vi "GUI_Final_PID.vi"() -> ()   [LabVIEW 2013]
uses:
  <vilib>/Instr/_visa.llb/VISA Configure Serial Port (Instr).vi
panel:
  in  "Send to encoder":bool
  out "Angle":u8[](array[numeric])
  out "Left":bool
  out "Right":bool
  out "read buffer":string
  in  "Stop":bool
  in  "Angle":string
  out "Error":errorcluster
  out "Arduino Data":string
  in  "Mode":bool
  in  "Baud Rate 2":u32=9600
  in  "Port 2":refnum<visa-resource-name>
  in  "Baud Rate":u32=9600
  in  "Port":refnum<visa-resource-name>
  out "Response 2":string
  in  "Command":string
  out "error out":errorcluster
  out "Numeric 12":i32
  in  "angle":i32
  in  "OK":bool
  in  "Commands":string(combo)
  out "error out 2":errorcluster
  in  "MODE":bool
  # "Arduino Interface"
  # "Encoder Interface"
  # "Text Mode"
  # "Button Mode"
  # "Select : ON : Text Mode , \n              OFF : ButtonMode"
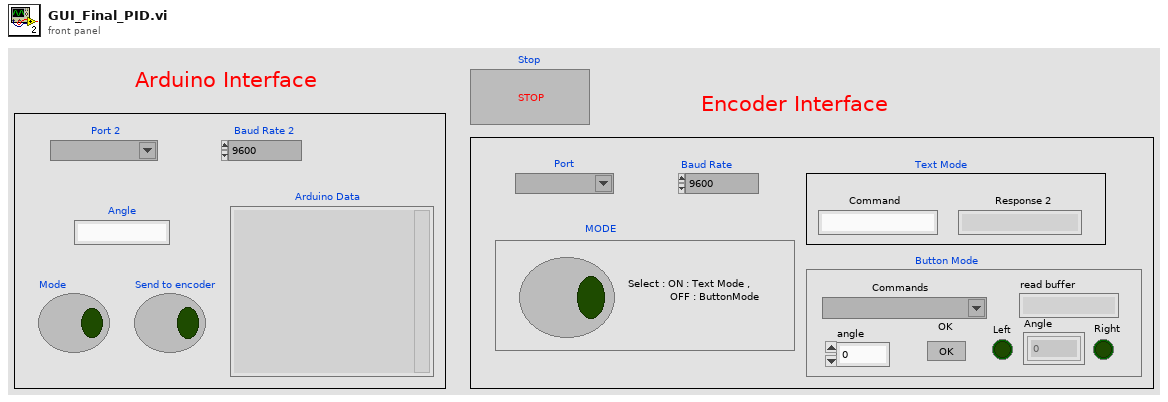
[diagram p1: front panel]
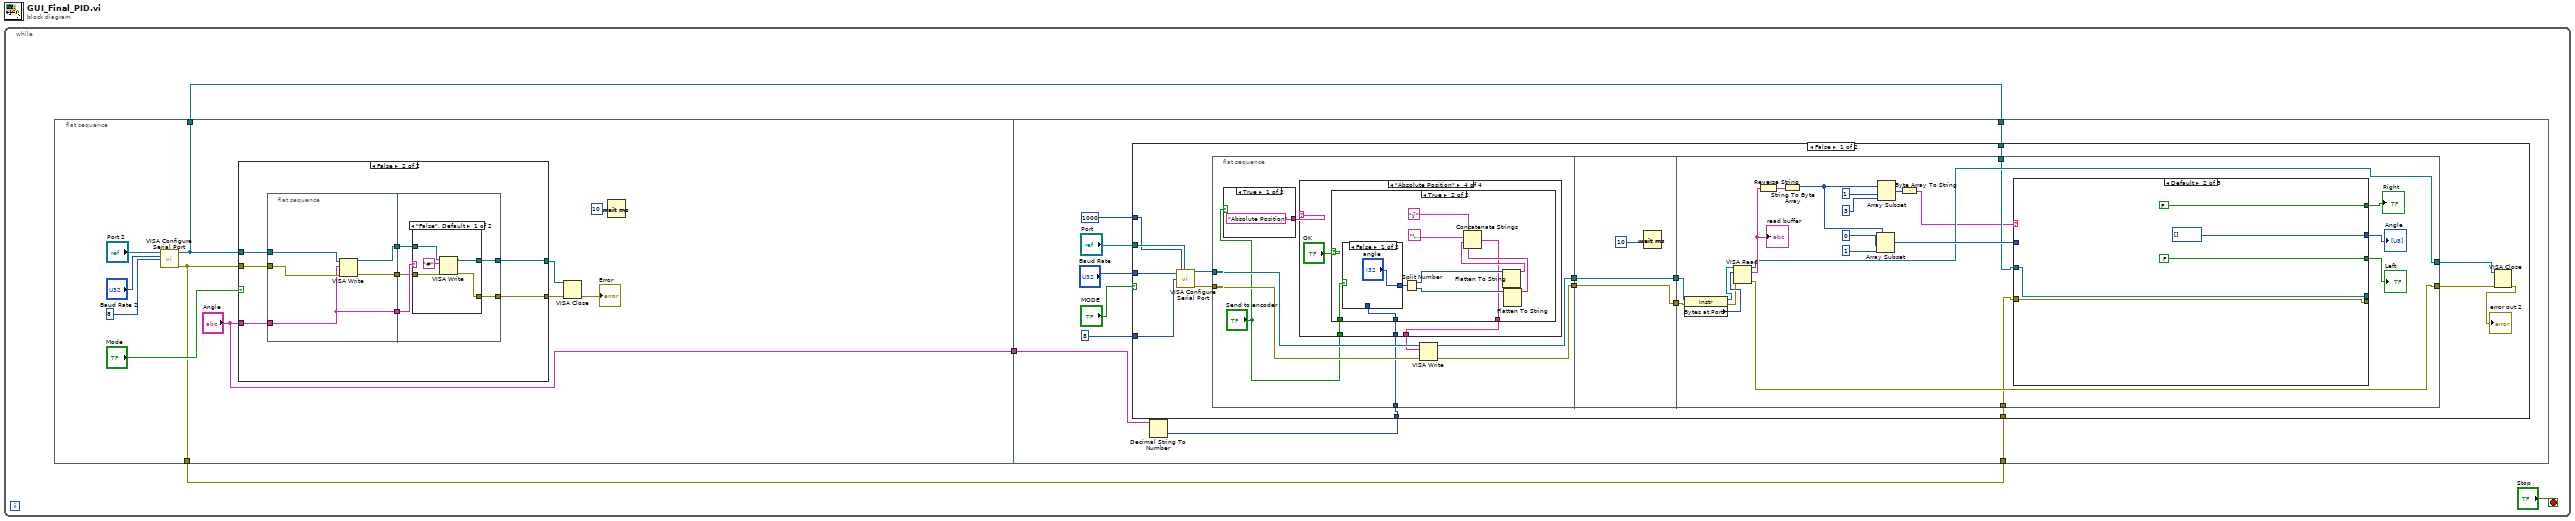
[diagram p0: block diagram]
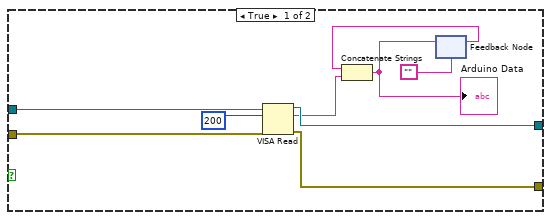
[diagram p2: hidden frame]
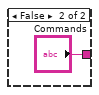
[diagram p4: hidden frame]
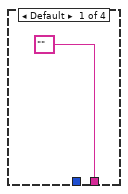
[diagram p5: hidden frame]
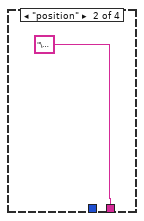
[diagram p6: hidden frame]
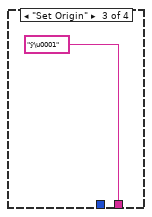
[diagram p7: hidden frame]
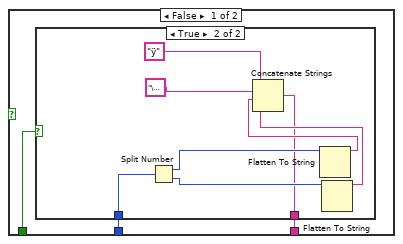
[diagram p8: hidden frame]
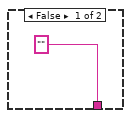
[diagram p9: hidden frame]
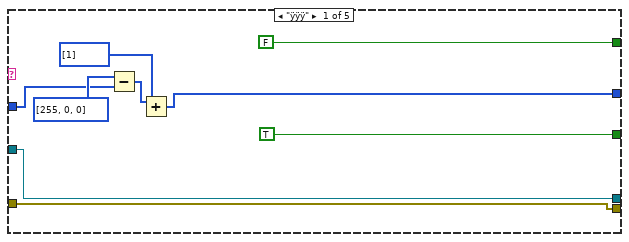
[diagram p11: hidden frame]
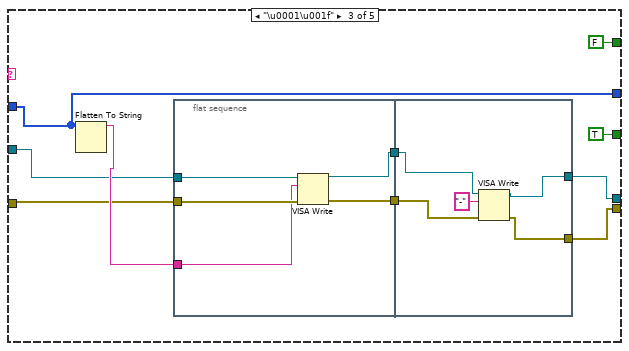
[diagram p12: hidden frame]
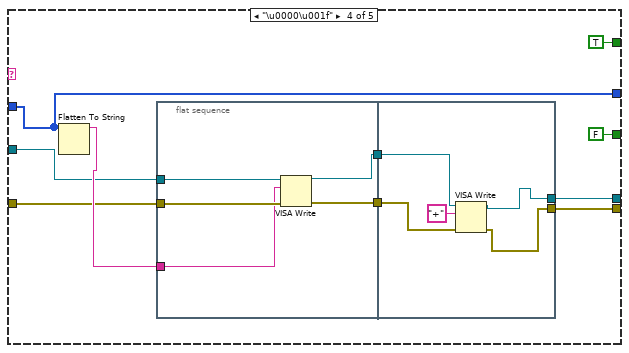
[diagram p13: hidden frame]
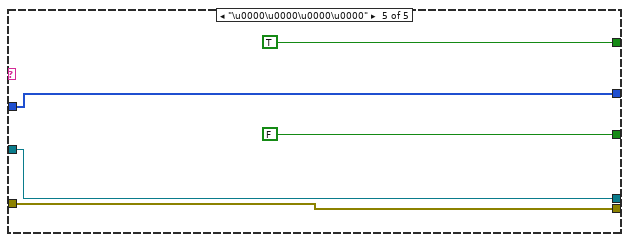
[diagram p14: hidden frame]
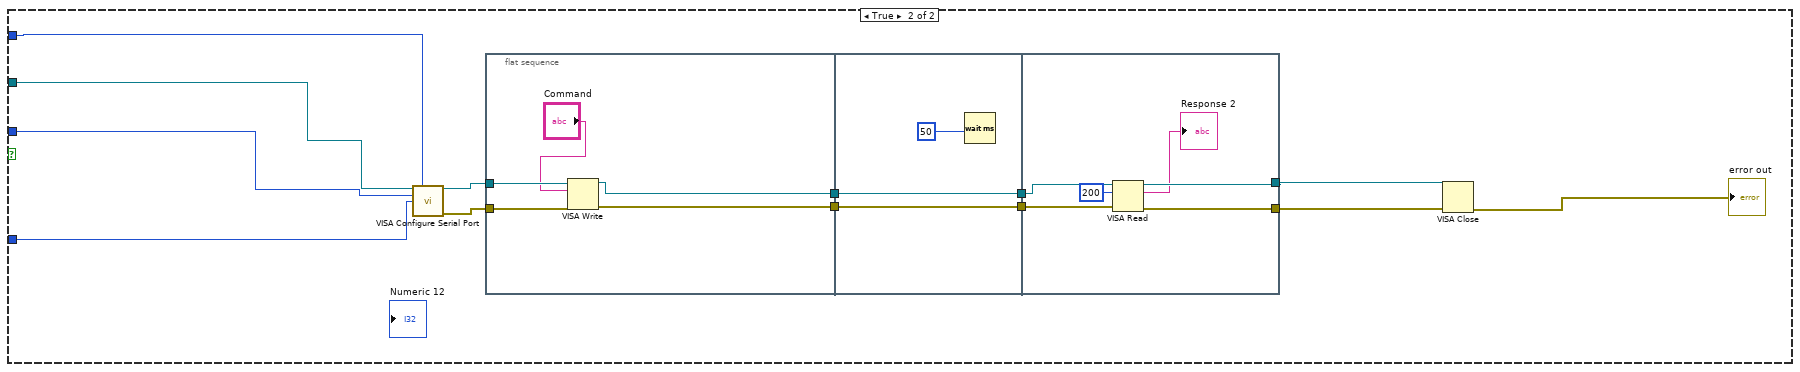
[diagram p15: hidden frame]
diagram:
  n1 = while {
    stop <- "Stop" stop-if-true
    n2 = flat-sequence {
      tunnel: ["Angle"] -> w4
      tunnel: [w6] -> w2
      tunnel: [w5] -> w1
      tunnel: w4 -> [w54]
      tunnel: w2 -> [w51]
      tunnel: w1 -> [w50]
      frame #0 {
        n3 = call-poly "VISA Configure Serial Port"("VISA resource name"="Port 2", "baud rate (9600)"="Baud Rate 2", "data bits (8)"=u16 8) -> ("VISA resource name out"=w6:refnum<visa-resource-name>, "error out"=w5:errorcluster)  [unwired: 11 in]
        n4 = case shown="False" "Mode" {
          tunnel: w6 -> [w22 w32]
          tunnel: [w23 w26] -> w14
          tunnel: [w24 w27] -> w15
          tunnel: w5 -> [w21 w31]
          tunnel: "Angle" -> [_ w25]
          frame True {
            n5 = VISA Read(VISA resource name=w22, byte count=u32 200, error in (no error)=w21) -> (VISA resource name out=w24:refnum<visa-resource-name>, read buffer=w19:string, error out=w23:errorcluster)  [unwired: 1 out]
            n6 = feedback #1("") -> (w18:string)
            n7 = Concatenate Strings(w18, w19) -> (w17:string)
            "Arduino Data" <- w17
            n8 = feedback-in #1(w17) -> ()
          }
          frame False {
            n9 = flat-sequence {
              tunnel: w32 -> [w37]
              tunnel: w31 -> [w36]
              tunnel: [w33] -> w30
              tunnel: [w35] -> w29
              tunnel: [w34] -> w28
              tunnel: w25 -> [w33]
              tunnel: w30 -> [w42]
              tunnel: w29 -> [w41]
              tunnel: w28 -> [w40]
              tunnel: [w39] -> w27
              tunnel: [w38] -> w26
              frame #0 {
                n10 = VISA Write(VISA resource name=w37, write buffer=w33, error in (no error)=w36) -> (VISA resource name out=w35:refnum<visa-resource-name>, error out=w34:errorcluster)  [unwired: 1 out]
              }
              frame #1 {
                n11 = case shown="\"False\", Default" w42 {
                  tunnel: w41 -> [w46 w49]
                  tunnel: w40 -> [w45 w48]
                  tunnel: [w44 w49] -> w39
                  tunnel: [w43 w48] -> w38
                  frame "False", Default {
                    n12 = VISA Write(VISA resource name=w46, write buffer="#", error in (no error)=w45) -> (VISA resource name out=w44:refnum<visa-resource-name>, error out=w43:errorcluster)  [unwired: 1 out]
                  }
                  frame "" {
                  }
                }
              }
            }
          }
        }
        n13 = VISA Close(VISA resource name=w15, error in (no error)=w14) -> (error out=→"Error":errorcluster)
        n14 = Wait (ms)(milliseconds to wait=u32 10) -> ()  [unwired: 1 out]
      }
      frame #1 {
        n15 = Decimal String To Number(string=w54) -> (number=w52:i32)  [unwired: 2 in, 1 out]
        n16 = case shown="False" "MODE" {
          tunnel: u32 1000 ("timeout (10sec)") -> [w63 w203]
          tunnel: "Port" -> [w68 w202]
          tunnel: "Baud Rate" -> [w67 w201]
          tunnel: u16 8 ("data bits (8)") -> [w65 w200]
          tunnel: w52 -> [w64 _]
          tunnel: w51 -> [w60 _]
          tunnel: w50 -> [w59 _]
          frame False {
            n17 = call-poly "VISA Configure Serial Port"("VISA resource name"=w68, "timeout (10sec)"=w63, "baud rate (9600)"=w67, "data bits (8)"=w65) -> ("VISA resource name out"=w72:refnum<visa-resource-name>, "error out"=w71:errorcluster)  [unwired: 10 in]
            n18 = flat-sequence {
              tunnel: [w81] -> w74
              tunnel: w72 -> [w80]
              tunnel: w71 -> [w79]
              tunnel: [w82] -> w70
              tunnel: w64 -> [w76]
              tunnel: [w117] -> w73
              tunnel: w74 -> [w116]
              tunnel: w70 -> [w117]
              tunnel: [w116] -> w69
              tunnel: w73 -> [w133]
              tunnel: w69 -> [w139]
              tunnel: [w123] -> w62
              tunnel: [w122] -> w61
              tunnel: w60 -> [w121]
              tunnel: w59 -> [w120]
              frame #0 {
                n19 = case shown="True" "Send to encoder" {
                  tunnel: ["Absolute Position" ("Commands") "Commands"] -> w78
                  frame True {
                  }
                  frame False {
                  }
                }
                n20 = case shown="\"Absolute Position\"" w78 {
                  tunnel: ["" "\u001f" "ÿ\u0001" w89] -> w77
                  tunnel: w76 -> [_ _ _ w90]
                  tunnel: "Send to encoder" -> [_ _ _ w88]
                  frame Default {
                  }
                  frame "position" {
                  }
                  frame "Set Origin" {
                  }
                  frame "Absolute Position" {
                    n21 = case shown="True" "OK" {
                      tunnel: w90 -> [w94 w105]
                      tunnel: [w93 w106] -> w89
                      tunnel: w88 -> [w92 w104]
                      frame False {
                        n22 = case shown="True" w92 {
                          tunnel: w94 -> [_ w97]
                          tunnel: ["" w96] -> w93
                          frame False {
                          }
                          frame True {
                            n23 = Split Number(x=w97) -> (hi(x)=w99:u16, lo(x)=w98:u16)
                            n24 = Flatten To String(anything=w99) -> (data string=w101:string)  [unwired: 3 in, 2 out]
                            n25 = Flatten To String(anything=w98) -> (data string=w100:string)  [unwired: 3 in, 2 out]
                            n26 = Concatenate Strings("ÿ" ("string"), "\u0002" ("string"), w101, w100) -> (w96:string)
                          }
                        }
                      }
                      frame True {
                        n27 = case shown="False" w104 {
                          tunnel: w105 -> [_ w115]
                          tunnel: ["angle" w115] -> w107
                          frame False {
                          }
                          frame True {
                          }
                        }
                        n28 = Split Number(x=w107) -> (hi(x)=w109:u16, lo(x)=w108:u16)
                        n29 = Flatten To String(anything=w109) -> (data string=w111:string)  [unwired: 3 in, 2 out]
                        n30 = Flatten To String(anything=w108) -> (data string=w110:string)  [unwired: 3 in, 2 out]
                        n31 = Concatenate Strings("ÿ" ("string"), "\u0002" ("string"), w111, w110) -> (w106:string)
                      }
                    }
                  }
                }
                n32 = VISA Write(VISA resource name=w80, write buffer=w77, error in (no error)=w79) -> (VISA resource name out=w82:refnum<visa-resource-name>, error out=w81:errorcluster)  [unwired: 1 out]
              }
              frame #1 {
                n33 = Wait (ms)(milliseconds to wait=u32 10) -> ()  [unwired: 1 out]
              }
              frame #2 {
                n34 = property class="Instr"(reference=w133, error in=w139) -> (reference out=w132:refnum<visa-resource-name>, error out=w138:errorcluster, "Bytes at Port"=w140:u32)
                n35 = VISA Read(VISA resource name=w132, byte count=w140, error in (no error)=w138) -> (VISA resource name out=w123:refnum<visa-resource-name>, read buffer=w135:string, error out=w122:errorcluster)  [unwired: 1 out]
                "read buffer" <- w135
                n36 = Reverse String(1:w135) -> (0:w131:string)
                n37 = String To Byte Array(string=w131) -> (unsigned byte array=w137:u8[])
                n38 = Array Subset(array=w137, index=0, length=1) -> (w124:u8[])
                n39 = Array Subset(array=w137, index=1, length=3) -> (w134:u8[])
                n40 = Byte Array To String(unsigned byte array=w134) -> (string=w119:string)
                n41 = case shown="Default" w119 {
                  tunnel: [w146 u8[] [] w155 w175 w195] -> w126
                  tunnel: [TRUE ("Boolean") FALSE ("Boolean") TRUE ("Boolean") FALSE ("Boolean") FALSE ("Boolean")] -> w125
                  tunnel: [FALSE ("Boolean") FALSE ("Boolean") FALSE ("Boolean") TRUE ("Boolean") TRUE ("Boolean")] -> w127
                  tunnel: w120 -> [w143 w151 w158 w179 w197]
                  tunnel: [w142 w150 w157 w178 w196] -> _
                  tunnel: [w143 w151 w156 w177 w197] -> _
                  tunnel: w121 -> [w142 w150 w159 w176 w196]
                  tunnel: w124 -> [w141 _ w155 w175 w195]
                  frame "ÿÿÿ" {
                    n42 = Subtract(x=u8[] [255, 0, 0] ("y"), y=w141) -> (x-y=w149:u8[])
                    n43 = Add(x=w149, y=u8[] [1]) -> (x+y=w146:u8[])
                  }
                  frame Default {
                  }
                  frame "\u0001\u001f" {
                    n44 = Flatten To String(anything=w155) -> (data string=w160:string)  [unwired: 3 in, 2 out]
                    n45 = flat-sequence {
                      tunnel: [w169] -> w162
                      tunnel: [w168] -> w161
                      tunnel: w159 -> [w167]
                      tunnel: w158 -> [w166]
                      tunnel: w160 -> [w165]
                      tunnel: w162 -> [w173]
                      tunnel: w161 -> [w172]
                      tunnel: [w171] -> w157
                      tunnel: [w170] -> w156
                      frame #0 {
                        n46 = VISA Write(VISA resource name=w167, write buffer=w165, error in (no error)=w166) -> (VISA resource name out=w169:refnum<visa-resource-name>, error out=w168:errorcluster)  [unwired: 1 out]
                      }
                      frame #1 {
                        n47 = VISA Write(VISA resource name=w173, write buffer="-", error in (no error)=w172) -> (VISA resource name out=w171:refnum<visa-resource-name>, error out=w170:errorcluster)  [unwired: 1 out]
                      }
                    }
                  }
                  frame "\u0000\u001f" {
                    n48 = Flatten To String(anything=w175) -> (data string=w180:string)  [unwired: 3 in, 2 out]
                    n49 = flat-sequence {
                      tunnel: [w189] -> w182
                      tunnel: [w188] -> w181
                      tunnel: w176 -> [w187]
                      tunnel: w179 -> [w186]
                      tunnel: w180 -> [w185]
                      tunnel: w182 -> [w192]
                      tunnel: w181 -> [w193]
                      tunnel: [w191] -> w178
                      tunnel: [w190] -> w177
                      frame #0 {
                        n50 = VISA Write(VISA resource name=w187, write buffer=w185, error in (no error)=w186) -> (VISA resource name out=w189:refnum<visa-resource-name>, error out=w188:errorcluster)  [unwired: 1 out]
                      }
                      frame #1 {
                        n51 = VISA Write(VISA resource name=w192, write buffer="+", error in (no error)=w193) -> (VISA resource name out=w191:refnum<visa-resource-name>, error out=w190:errorcluster)  [unwired: 1 out]
                      }
                    }
                  }
                  frame "\u0000\u0000\u0000\u0000" {
                  }
                }
                "Left" <- w125
                "Right" <- w127
                "Angle" <- w126
              }
            }
            n52 = VISA Close(VISA resource name=w62, error in (no error)=w61) -> (error out=→"error out 2":errorcluster)
          }
          frame True {
            n53 = call-poly "VISA Configure Serial Port"("VISA resource name"=w202, "timeout (10sec)"=w203, "baud rate (9600)"=w201, "data bits (8)"=w200) -> ("VISA resource name out"=w208:refnum<visa-resource-name>, "error out"=w207:errorcluster)  [unwired: 10 in]
            n54 = flat-sequence {
              tunnel: w208 -> [w215]
              tunnel: w207 -> [w217]
              tunnel: [w214] -> w212
              tunnel: [w216] -> w211
              tunnel: [w219] -> w210
              tunnel: w212 -> [w219]
              tunnel: [w218] -> w209
              tunnel: w211 -> [w218]
              tunnel: w210 -> [w226]
              tunnel: w209 -> [w225]
              tunnel: [w224] -> w205
              tunnel: [w223] -> w206
              frame #0 {
                n55 = VISA Write(VISA resource name=w215, write buffer="Command", error in (no error)=w217) -> (VISA resource name out=w214:refnum<visa-resource-name>, error out=w216:errorcluster)  [unwired: 1 out]
              }
              frame #1 {
                n56 = Wait (ms)(milliseconds to wait=u32 50) -> ()  [unwired: 1 out]
              }
              frame #2 {
                n57 = VISA Read(VISA resource name=w226, byte count=u32 200, error in (no error)=w225) -> (VISA resource name out=w223:refnum<visa-resource-name>, read buffer=→"Response 2":string, error out=w224:errorcluster)  [unwired: 1 out]
              }
            }
            n58 = VISA Close(VISA resource name=w206, error in (no error)=w205) -> (error out=→"error out":errorcluster)
          }
        }
      }
    }
  }
